vi "desc sort selected columns.vi"(1 "disabled index (col)":i32, 2 "all rows in":dbl[][](array[numeric])) -> (0 "1d sorted array (desc)":dbl[](array[numeric]))   [LabVIEW 2023]
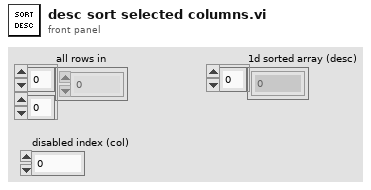
[diagram p1: front panel]
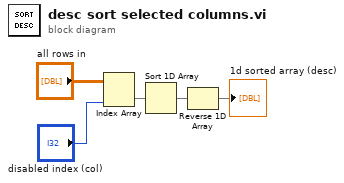
[diagram p0: block diagram]
diagram:
  n1 = Index Array(array="all rows in", index (col)="disabled index (col)") -> (element=w4:dbl[])  [unwired: 1 in]
  n2 = Sort 1D Array(array=w4) -> (sorted array=w1:dbl[])
  n3 = Reverse 1D Array(array=w1) -> (reversed array=→"1d sorted array (desc)":dbl[])
